vi "Results User Event LV2.vi"(0 "user event":refnum<user-event>, 11 "error in (no error)":errorcluster, 13 "LV2 operations":enum16{"Read", "Write"}(ring)) -> (4 "user event out":refnum<user-event>, 15 "error out":errorcluster)   [LabVIEW 2021]
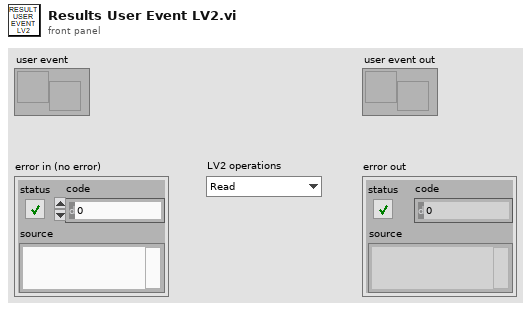
[diagram p1: front panel]
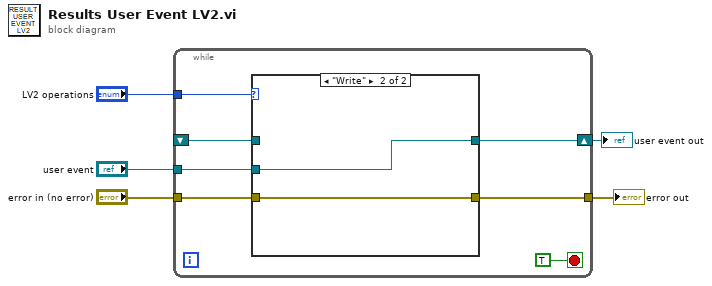
[diagram p0: block diagram]
diagram:
  n1 = while {
    tunnel: "LV2 operations" -> [w11]
    tunnel: "error in (no error)" -> [w10]
    tunnel: [w9] -> w3
    shift-right: [w7] -> w1
    shift-left: _ -> [w6]
    tunnel: "user event" -> [w8]
    stop <- TRUE stop-if-true
    n2 = case shown="\"Write\"" w11 {
      tunnel: w10 -> [w13 w16]
      tunnel: [w13 w16] -> w9
      tunnel: w8 -> [_ w15]
      tunnel: [w14 w15] -> w7
      tunnel: w6 -> [w14 _]
      frame "Read", Default {
      }
      frame "Write" {
      }
    }
  }
  "error out" <- w3
  "user event out" <- w1
